vi "WriteDigitalOutput.vi"(8 "error in (no error)":errorcluster, 9 "Tristate":bool, 10 "data":bool, 11 "DigitalOutput_Simulation In":refnum<class "TesteractHAL_DigitalOutput_Simulation.lvclass">) -> (0 "error out":errorcluster, 3 "DigitalOutput_Simulation Out":refnum<class "TesteractHAL_DigitalOutput_Simulation.lvclass">)   [LabVIEW 2017, in "TesteractHAL_DigitalOutput_Simulation.lvlib" / "TesteractHAL_DigitalOutput_Simulation.lvclass"]
doc: "Write a single digital signal."
uses:
  TesteractHAL_DigitalOutput_Simulation.lvclass
  TesteractHAL_DigitalOutput_Simulation.lvclass/TesteractHAL_DigitalOutput_Simulation.ctl
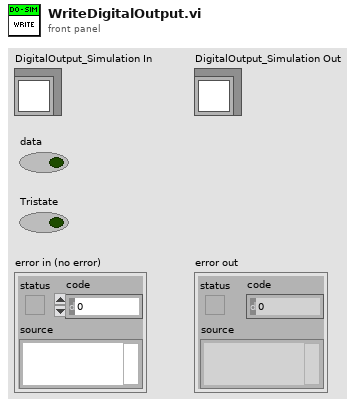
[diagram p1: front panel]
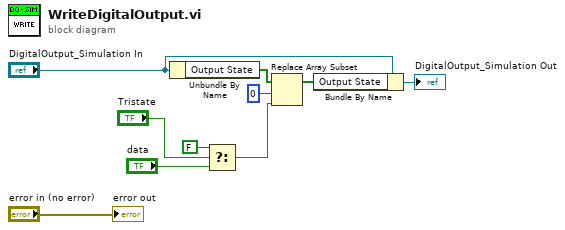
[diagram p0: block diagram]
diagram:
  n1 = Unbundle By Name("DigitalOutput_Simulation In") -> ("Output State"=w8:bool[])
  n2 = Select(t=FALSE, s="Tristate", f="data") -> (s? t:f=w1:bool)
  n3 = Replace Array Subset(array=w8, new element=w1, index=0) -> (w6:bool[])
  n4 = Bundle By Name(cluster="DigitalOutput_Simulation In", "Output State"=w6) -> (→"DigitalOutput_Simulation Out":refnum<class "TesteractHAL_DigitalOutput_Simulation.lvclass">)
  "error out" <- "error in (no error)"
